vi "Choreo_Util_AllianceFlipTranslation2d.vi"(11 "Translation":T1 {"Y" format="%14.3f"; "X" format="%14.3f"}) -> (3 "FlippedTranslation":T1 {"Y" format="%14.3f"; "X" format="%14.3f"})   [LabVIEW 2019, in "ChoreoLib.lvlib"]
doc: "Flips a translation2d cluster.\n\nInputs: \n -- translation - translation2d - The translation to flip.\n\nOutputs:\n -- FlippedTranslation - Translation2d - The flipped cluster"
uses:
  ChoreoLib.lvlib
  <vilib>/Rock Robotics/WPI/ThirdParty/JAS_Junk/TrajLib/TypeDef/TRANSLATION2D.ctl
  Choreo_Choreo_Globals.vi
  <vilib>/Rock Robotics/WPI/ThirdParty/JAS_Junk/TrajLib/Trajectory_Library.lvlib
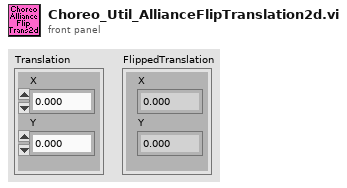
[diagram p1: front panel]
types:
  T1 = typedef "Trajectory_Library.lvlib/TRANSLATION2D.ctl" = cluster{"X":dbl, "Y":dbl}
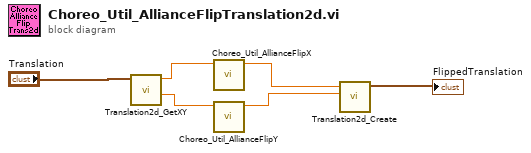
[diagram p0: block diagram]
diagram:
  n1 = call <vilib>:"Translation2d_GetXY.vi"("In Translation"="Translation") -> ("Y"=w3:dbl, "X"=w4:dbl)  [unwired: 9 in]
  n2 = call "Choreo_Util_AllianceFlipX.vi"("X"=w4) -> ("FlippedX"=w2:dbl)  [unwired: 10 in]
  n3 = call "Choreo_Util_AllianceFlipY.vi"("Y"=w3) -> ("FlippedY"=w1:dbl)  [unwired: 10 in]
  n4 = call <vilib>:"Translation2d_Create.vi"("Y"=w1, "X"=w2) -> ("TRANSLATION"=→"FlippedTranslation":T1)  [unwired: 9 in]
